vi "PKYK_Serial_No.vi"(11 "Strings []":string[](array[string])) -> (3 "Serial Number":string)   [LabVIEW 2020]
uses:
  <userlib>/_OpenG.lib/array/array.llb/Filter 1D Array (I32)__ogtk.vi
panel:
  out "min value":i32
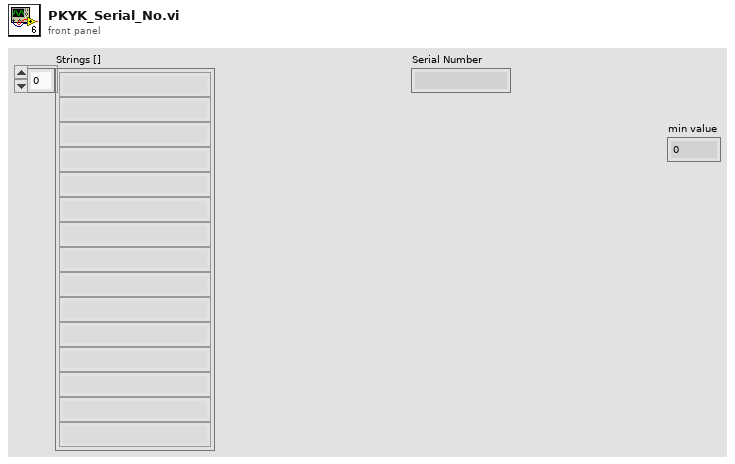
[diagram p1: front panel]
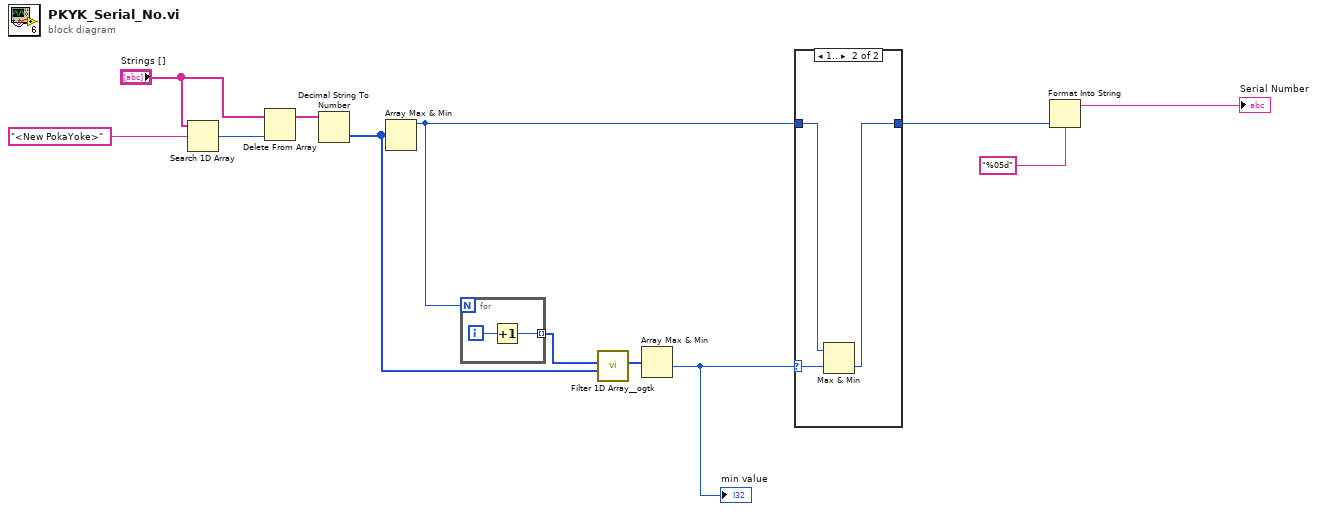
[diagram p0: block diagram]
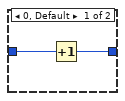
[diagram p2: hidden frame]
diagram:
  n1 = Search 1D Array(1D array="Strings []", element="<New PokaYoke>") -> (index of element=w9:i32)  [unwired: 1 in]
  n2 = Delete From Array(array="Strings []", index=w9) -> (array with subset deleted=w7:string[])  [unwired: 1 in, 1 out]
  n3 = Decimal String To Number(string=w7) -> (number=w5:i32[])  [unwired: 2 in, 1 out]
  n4 = Array Max & Min(array=w5) -> (max value=w2:i32)  [unwired: 3 out]
  n5 = for {
    N: w2 -> [_]
    tunnel: [w13] -> w6 mode=indexing
    i -> [w14]
    n6 = Increment(x=w14) -> (x+1=w13:i32)
  }
  n7 = call-poly <userlib>:"Filter 1D Array__ogtk.vi"("items to filter"=w5, "array"=w6) -> ("filtered array"=w4:i32[])  [unwired: 4 in, 1 out]
  n8 = Array Max & Min(array=w4) -> (min value=w3:i32)  [unwired: 3 out]
  "min value" <- w3
  n9 = case shown="1.." w3 {
    selector: w3 -> [_ w19]
    tunnel: w2 -> [w16 w18]
    tunnel: [w15 w17] -> w1
    frame 0, Default {
      n10 = Increment(x=w16) -> (x+1=w15:i32)
    }
    frame 1.. {
      n11 = Max & Min(x=w18, y=w19) -> (min(x,y)=w17:i32)  [unwired: 1 out]
    }
  }
  n12 = Format Into String(format string="%05d", w1) -> (resulting string=→"Serial Number":string)  [unwired: 2 in, 1 out]
